vi "Reset Branch Status.vi"(8 "error in (no error)":errorcluster, 11 "bt_Parallel in":refnum<class "bt_Parallel.lvclass">) -> (0 "error out":errorcluster, 3 "bt_Parallel out":refnum<class "bt_Parallel.lvclass">)   [LabVIEW 2021, in "BT.lvlib" / "bt_Parallel.lvclass"]
uses:
  bt_Parallel.lvclass
  bt_Parallel.lvclass/bt_Parallel.ctl
  abs_Node/Status.ctl
  abs_Node/bt_Node.lvclass
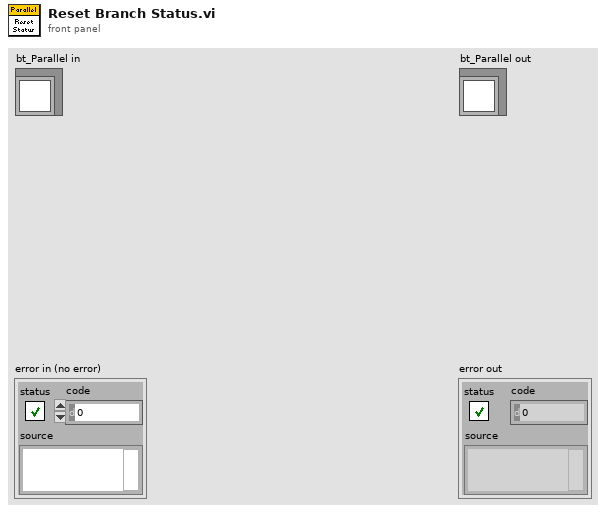
[diagram p1: front panel]
types:
  T1 = typedef "BT.lvlib/bt_Node.lvclass/Status.ctl" = enum16{"Success", "Failure", "Running"}
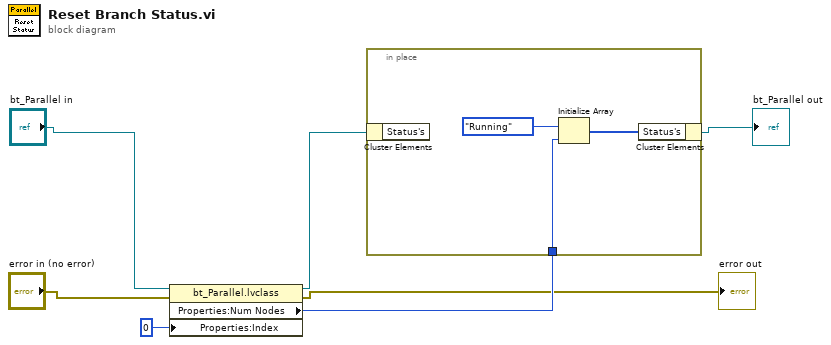
[diagram p0: block diagram]
diagram:
  n1 = property class="bt_Parallel.lvclass"(reference="bt_Parallel in", error in="error in (no error)", "Properties:Index"=0 ("Index")) -> (reference out=w4:refnum<class "bt_Parallel.lvclass">, error out=→"error out":errorcluster, "Properties:Num Nodes"=w3:i32)
  n2 = in-place {
    in-place-border: w3 -> [w8]
    n3 = in-place-cluster #1(w4) -> ()  [unwired: 1 out]
    n4 = Initialize Array(Status."Running" ("Status"), w8) -> (w9:T1[])
    n5 = in-place-cluster #1("Status's"=w9) -> (→"bt_Parallel out":refnum<class "bt_Parallel.lvclass">)
  }
